vi "Run.vi"(8 "error in (no error)":errorcluster, 11 "IMD in":refnum<class "IMD.lvclass">) -> (0 "error out":errorcluster, 1 "Parameters":cluster{"Name":string, "Value":string}[](array[cluster]), 2 "Cancled":bool, 3 "IMD out":refnum<class "IMD.lvclass">)   [LabVIEW 2020, in "IMD.lvclass"]
doc: "This is the main test vi. It is here that the test is implemented."
uses:
  IMD.lvclass
  C:/Sandbox/RF Bench/Source Code/WiSpry Test Framework/Measurements/Measurement.lvclass
  Controls/Run states.ctl
  Devices/Controls/Change setting mode enum.ctl
  IMD.lvclass/IMD.ctl
  Instruments/Spectrum Analyzer/Spectrum Analyzer.lvclass/Spectrum Analyzer.ctl
  Measurement.lvclass/Measurement.ctl
  Path Control/Paths.ctl
  Support VI/Update parameters (single).vi
  Support VI/Update parameters (array).vi
  Measurement.lvclass
  Devices/Device.lvclass
  Instruments/Signal Generator/Signal Generator.lvclass
  Instruments/Spectrum Analyzer/Spectrum Analyzer.lvclass
  Devices/PIC-device/PIC-Device.lvclass
  XML Handler/XML Handler.lvclass
  Path Control/PathControl.lvclass
panel:
  in  "Power readings":dbl[](array[numeric])
  out "Current Delta Power [dB]":dbl
  out "Device Parameters":string
  out "Current Offset [Hz]":dbl format="%#_6p"
  out "Current Power [dBm]":dbl
  out "Current Frequency [Hz]":dbl format="%#_6p"
  out "Progress":u8(slide) scale=0.0..100.0
  in  "Cancel Button":bool
  out "XY Graph":cluster{dbl[], dbl[]}[](graph)
  out "Estimated finish time":timestamp format="%<%X>T"
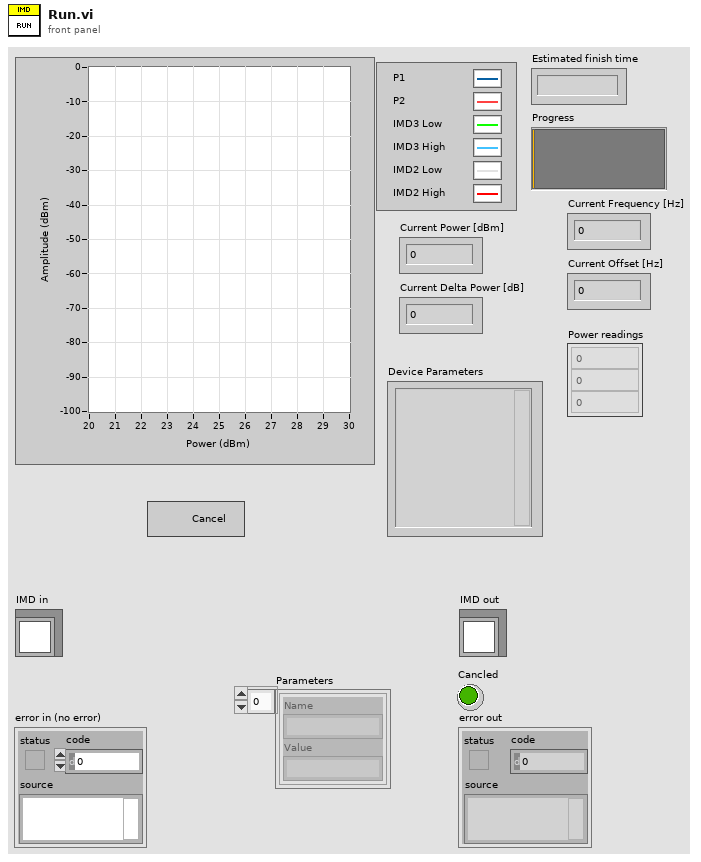
[diagram p1: front panel]
types:
  T1 = typedef "IMD.lvclass/Run states.ctl" = enum16{"Init", "Set Device", "Set Power", "Set Delta Power", "Set Frequency", "Set Offset", "Measure", "Done"}
  T2 = enum32{"Invalid", "Standard", "Closed", "Hidden", "Minimized", "Maximized"}
  T3 = typedef "PIC-Device.lvclass/Change setting mode enum.ctl" = enum16{"Init", "Next", "Reset"}
  T4 = typedef "IMD.lvclass/Config info.ctl" = cluster{"RBW":dbl, "VBW ":dbl, "Number of Averages":dbl, "Average On":bool, "Frequency (MHz)":string, "Offset Frequency (MHz)":string, "Power (dBm)":string, "Delta Power (dB)":string, "Uneven IMD":bool, "Loop order":T5, "Stop level":dbl, "IMD2":bool, "IMD3":bool}
  T5 = typedef "IMD.lvclass/Loop order.ctl" = enum16{"Device -> Power -> Frequency -> Offset", "Device -> Frequency -> Power -> Offset"}
  T6 = typedef "XML Handler.lvclass/Result Cluster.ctl" = cluster{"Name":string, "Value":string}
  T7 = typedef "PathControl.lvclass/Paths.ctl" = enum16{"SigGen 1 -> DUT", "SigGen 2 -> DUT", "SigGen 1 -> PM 1", "SigGen 1 -> PM 2", "DUT -> SA", "DUT -> PM 2", "VSG -> DUT", "SigGen 2 -> PM 1", "SigGen 2 -> PM 2"}
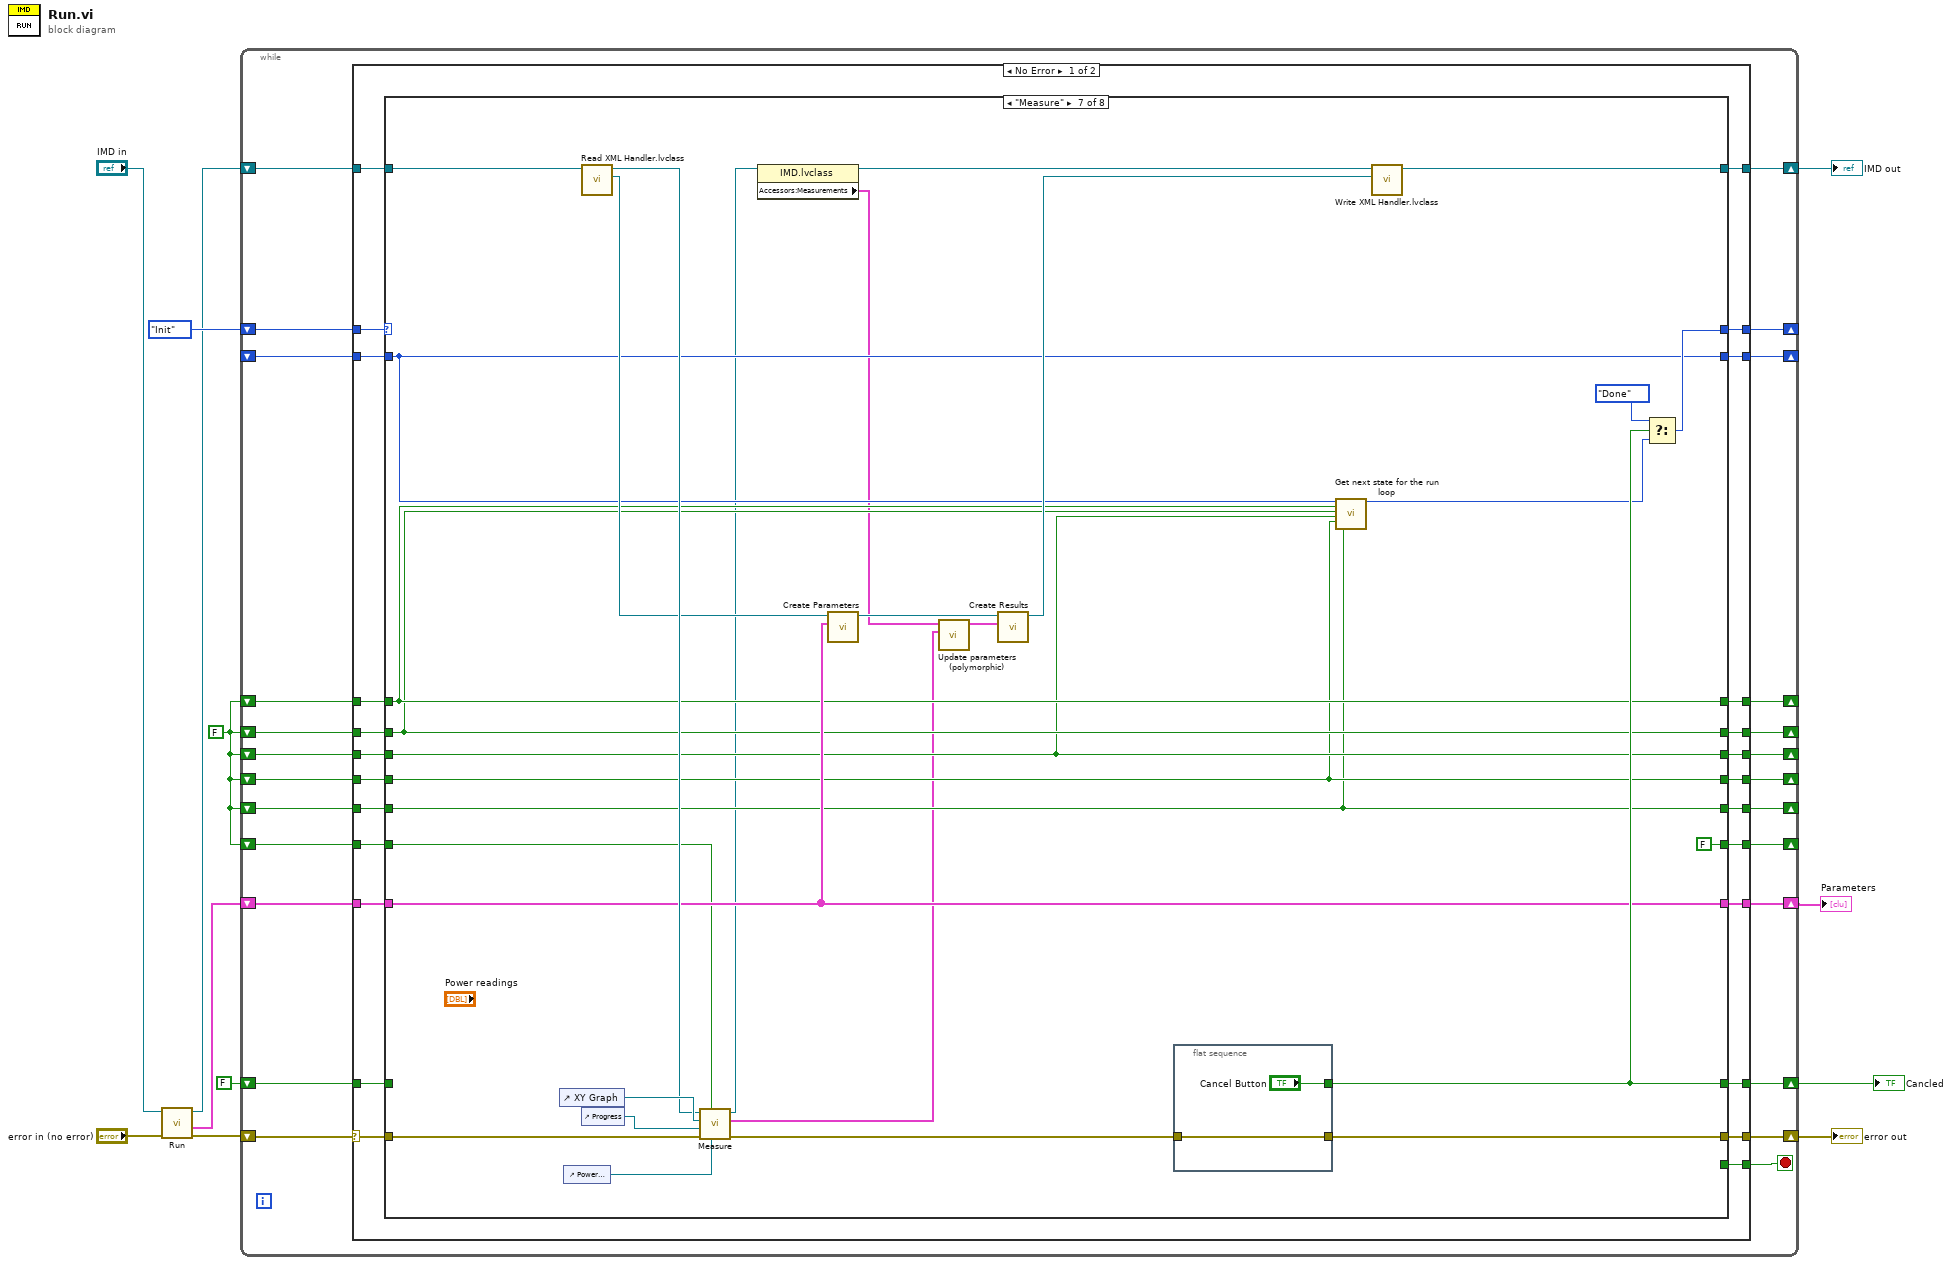
[diagram p0: block diagram]
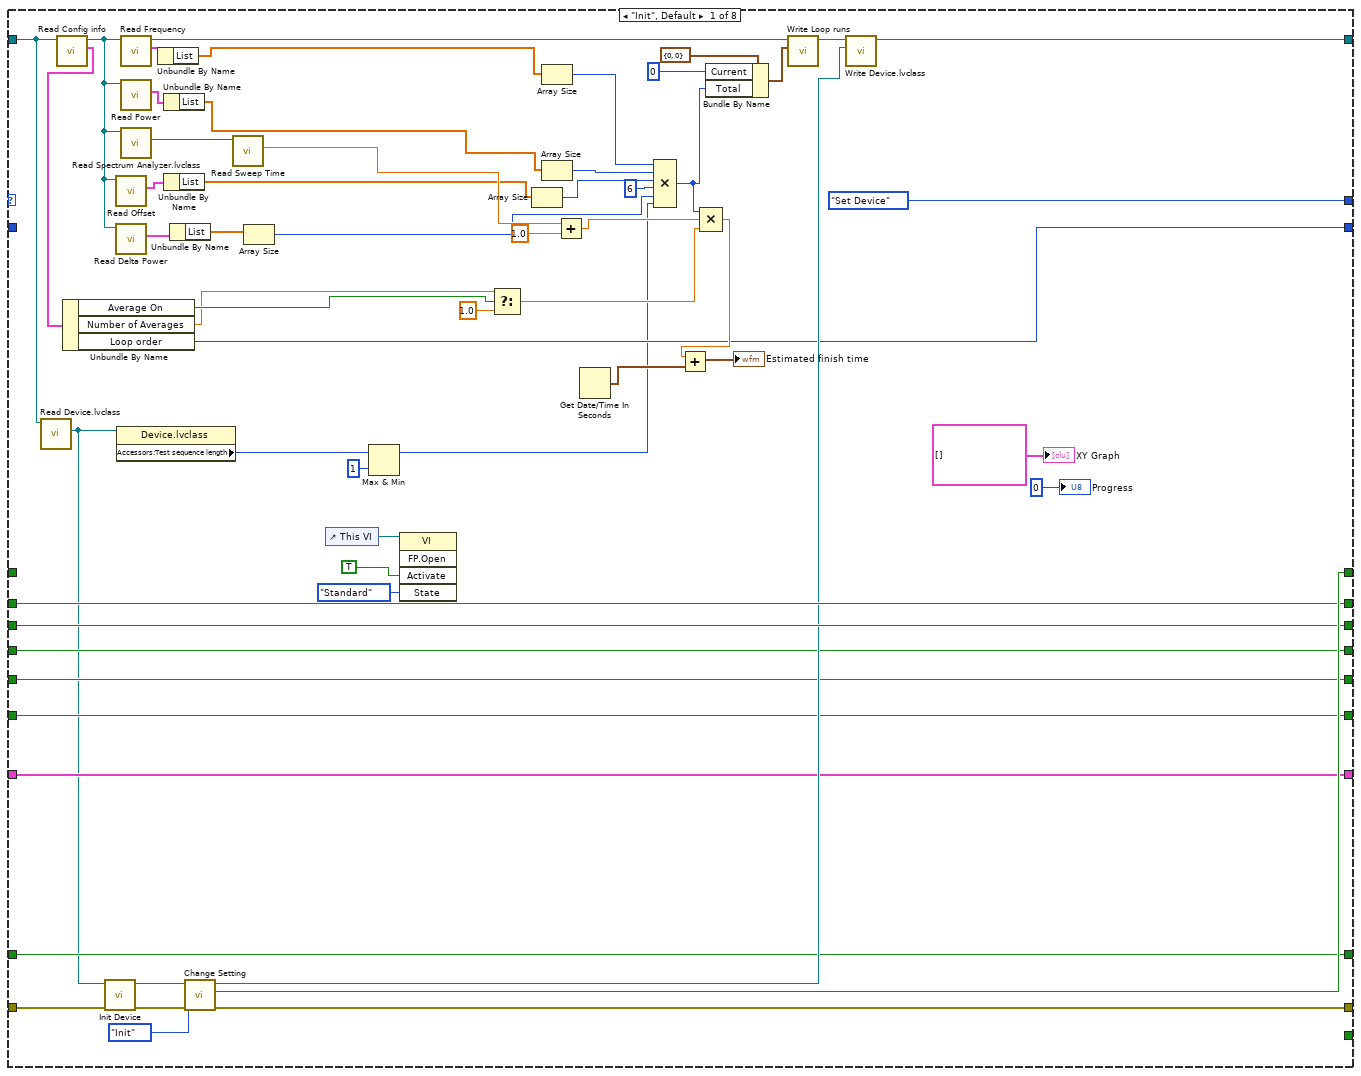
[diagram p2: hidden frame]
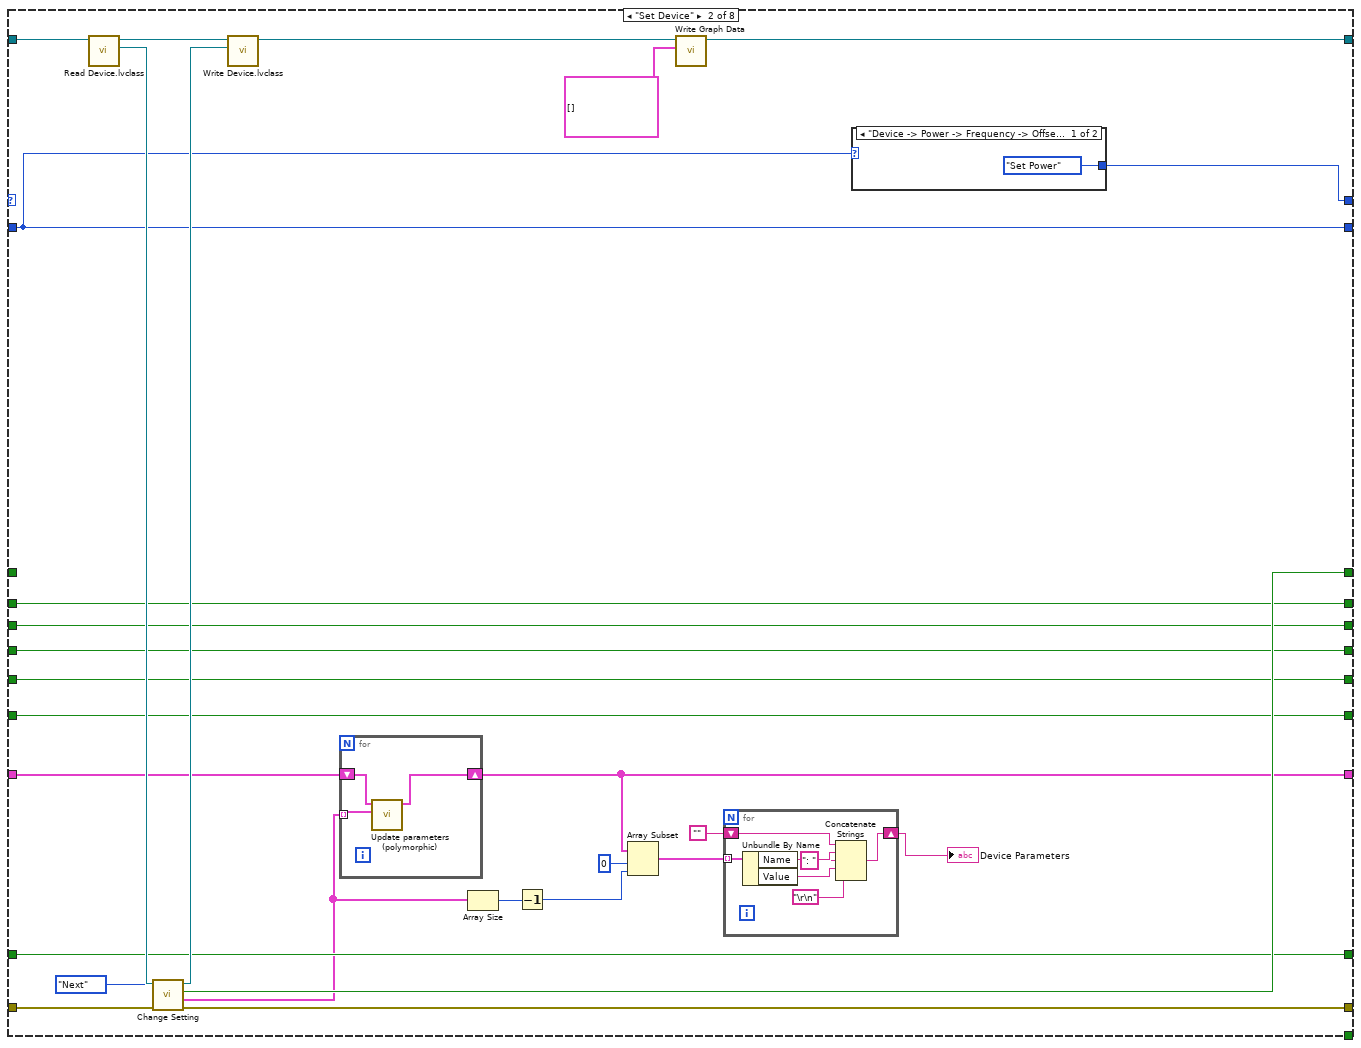
[diagram p3: hidden frame]
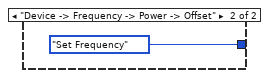
[diagram p4: hidden frame]
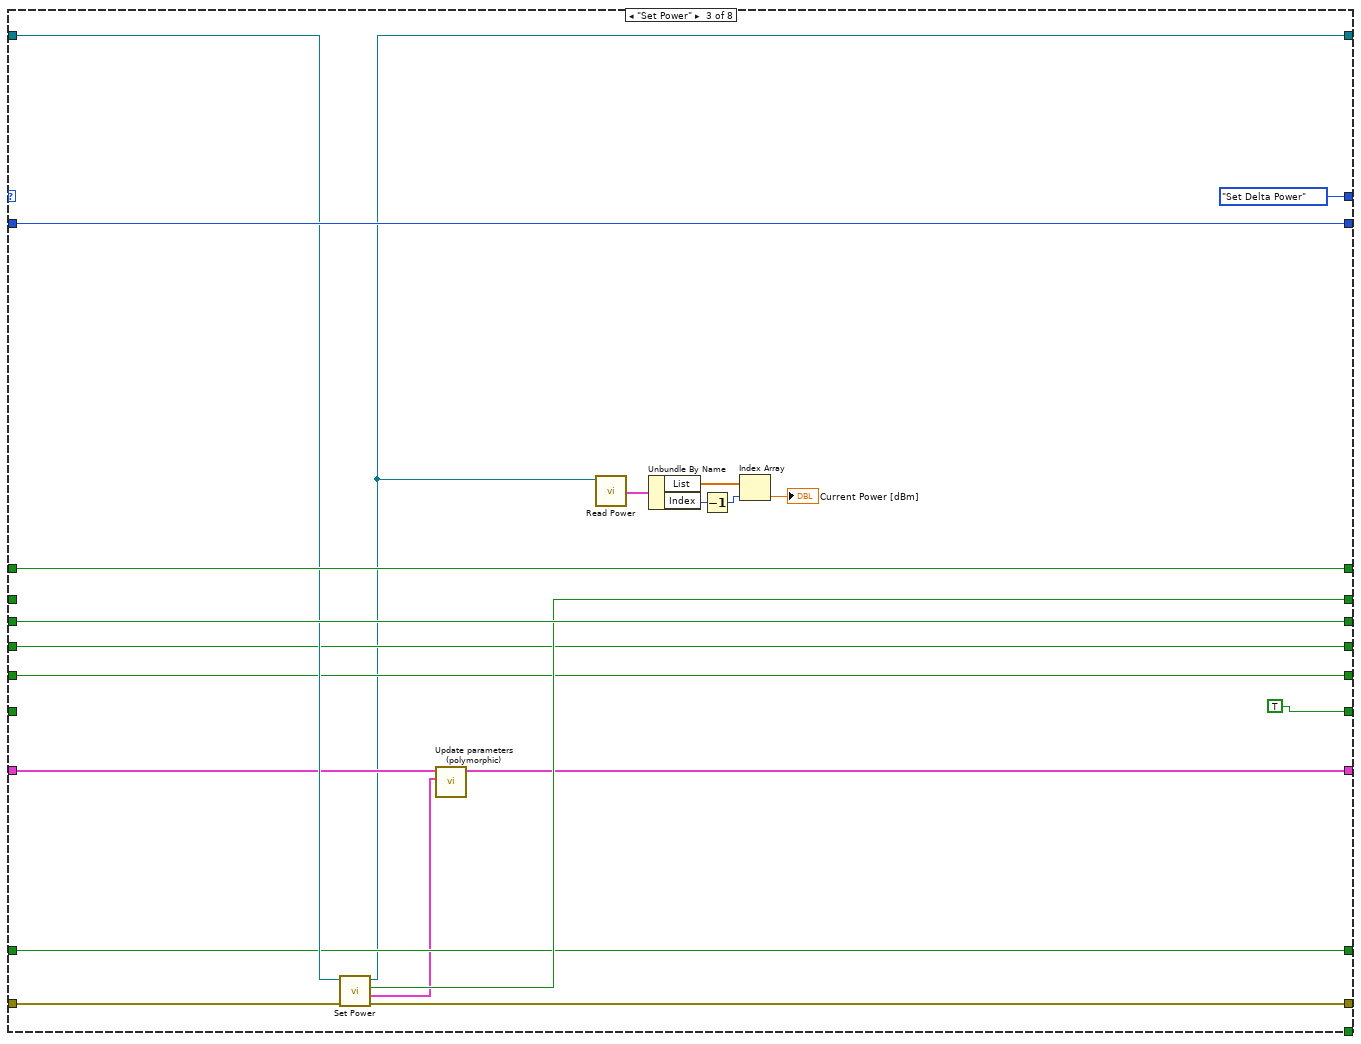
[diagram p5: hidden frame]
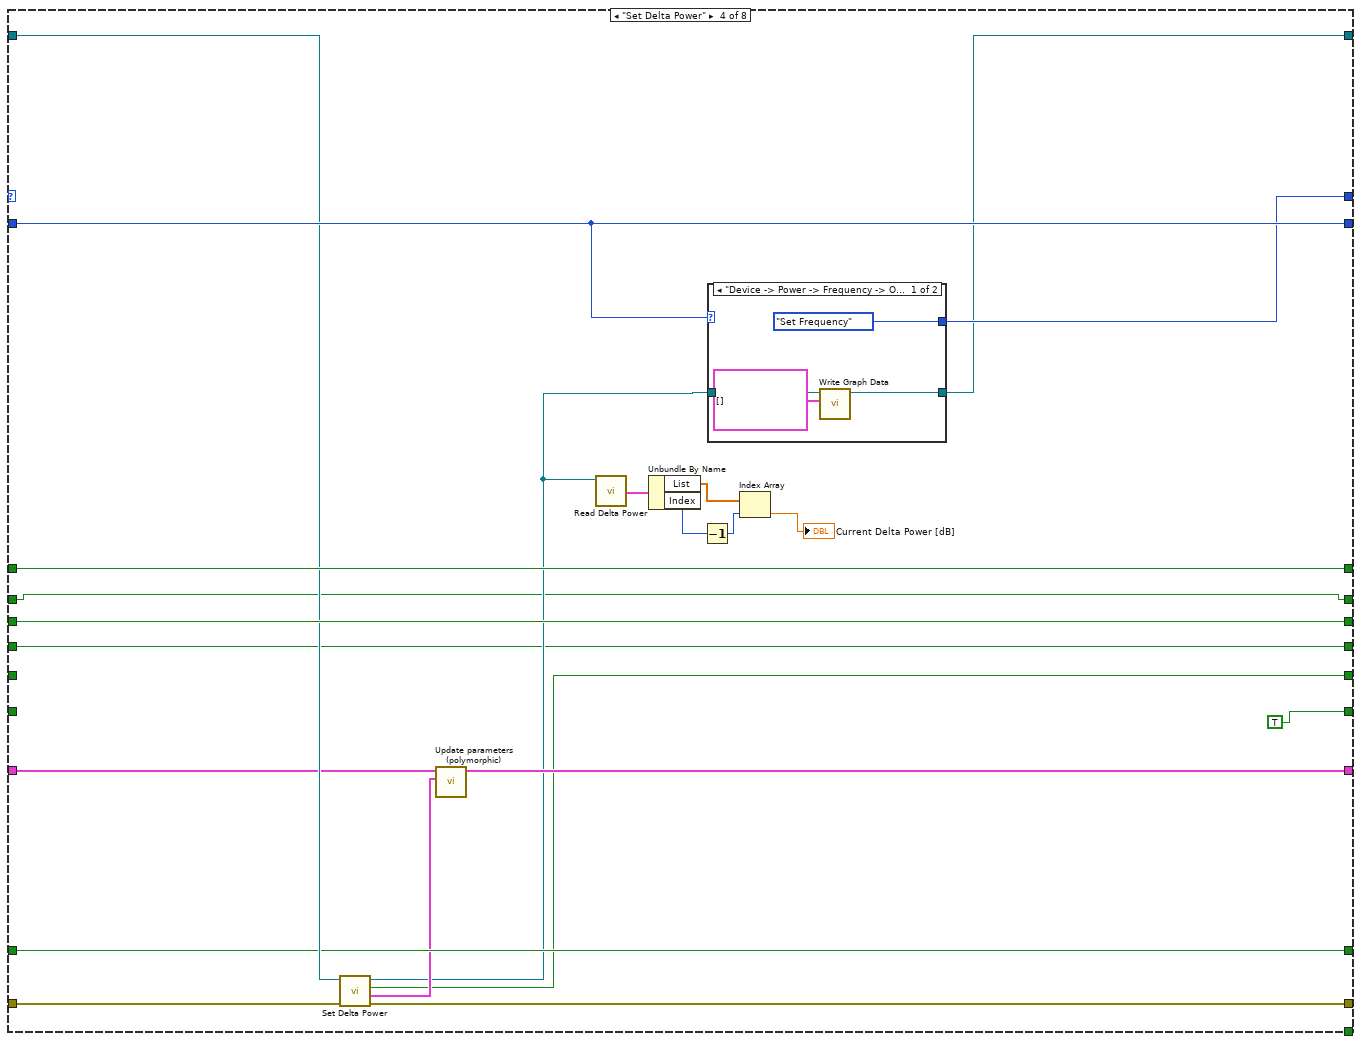
[diagram p6: hidden frame]
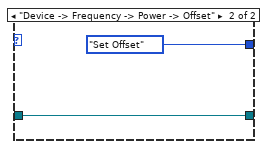
[diagram p7: hidden frame]
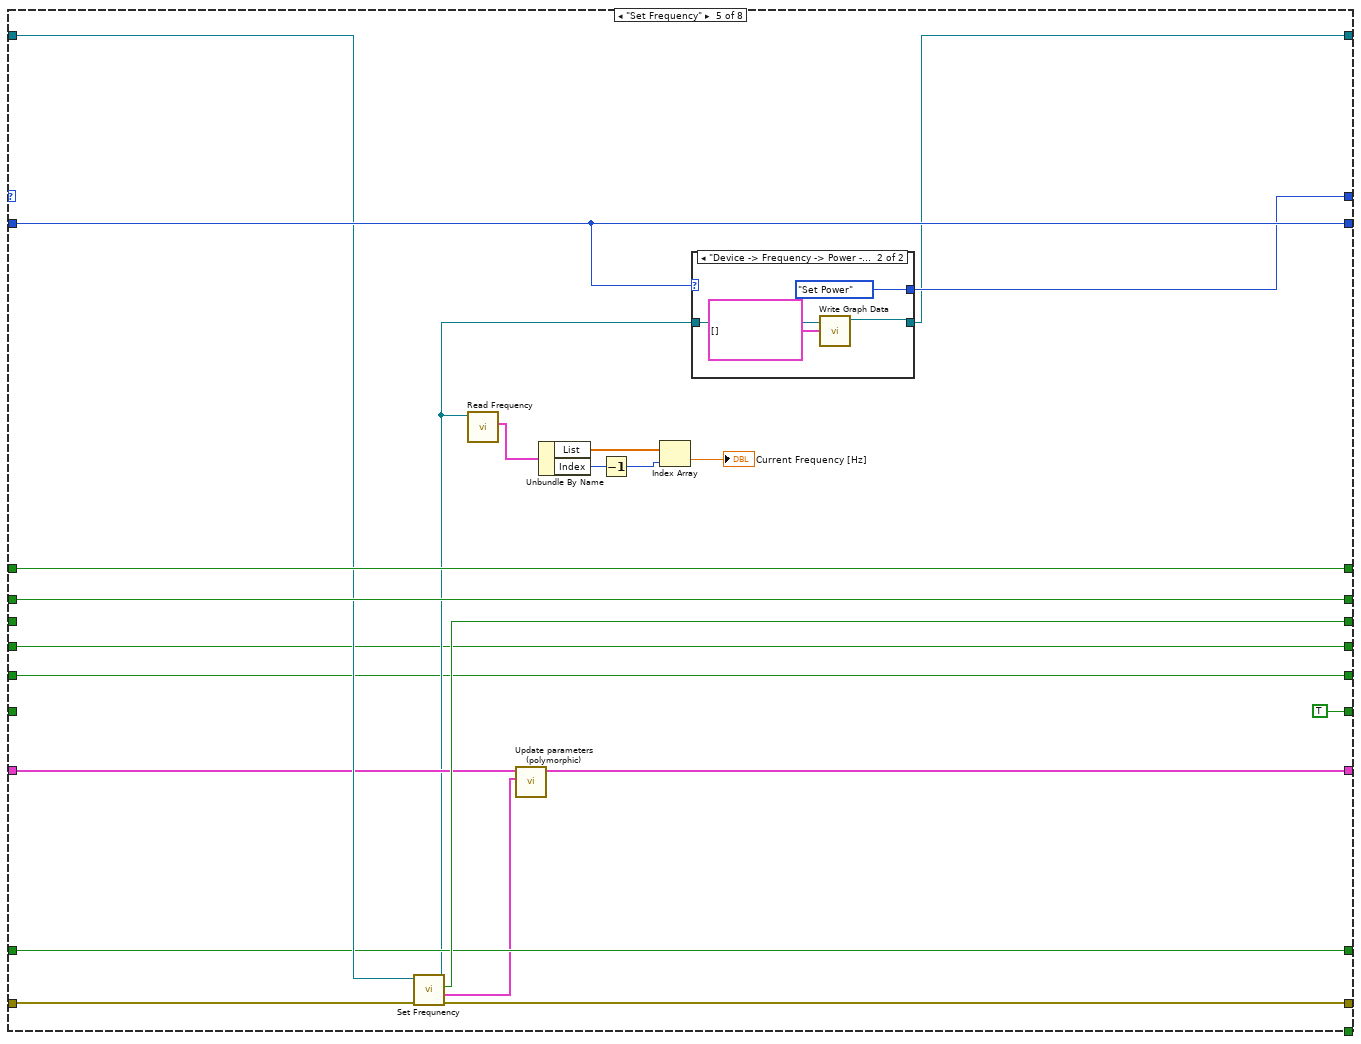
[diagram p8: hidden frame]
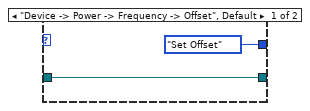
[diagram p9: hidden frame]
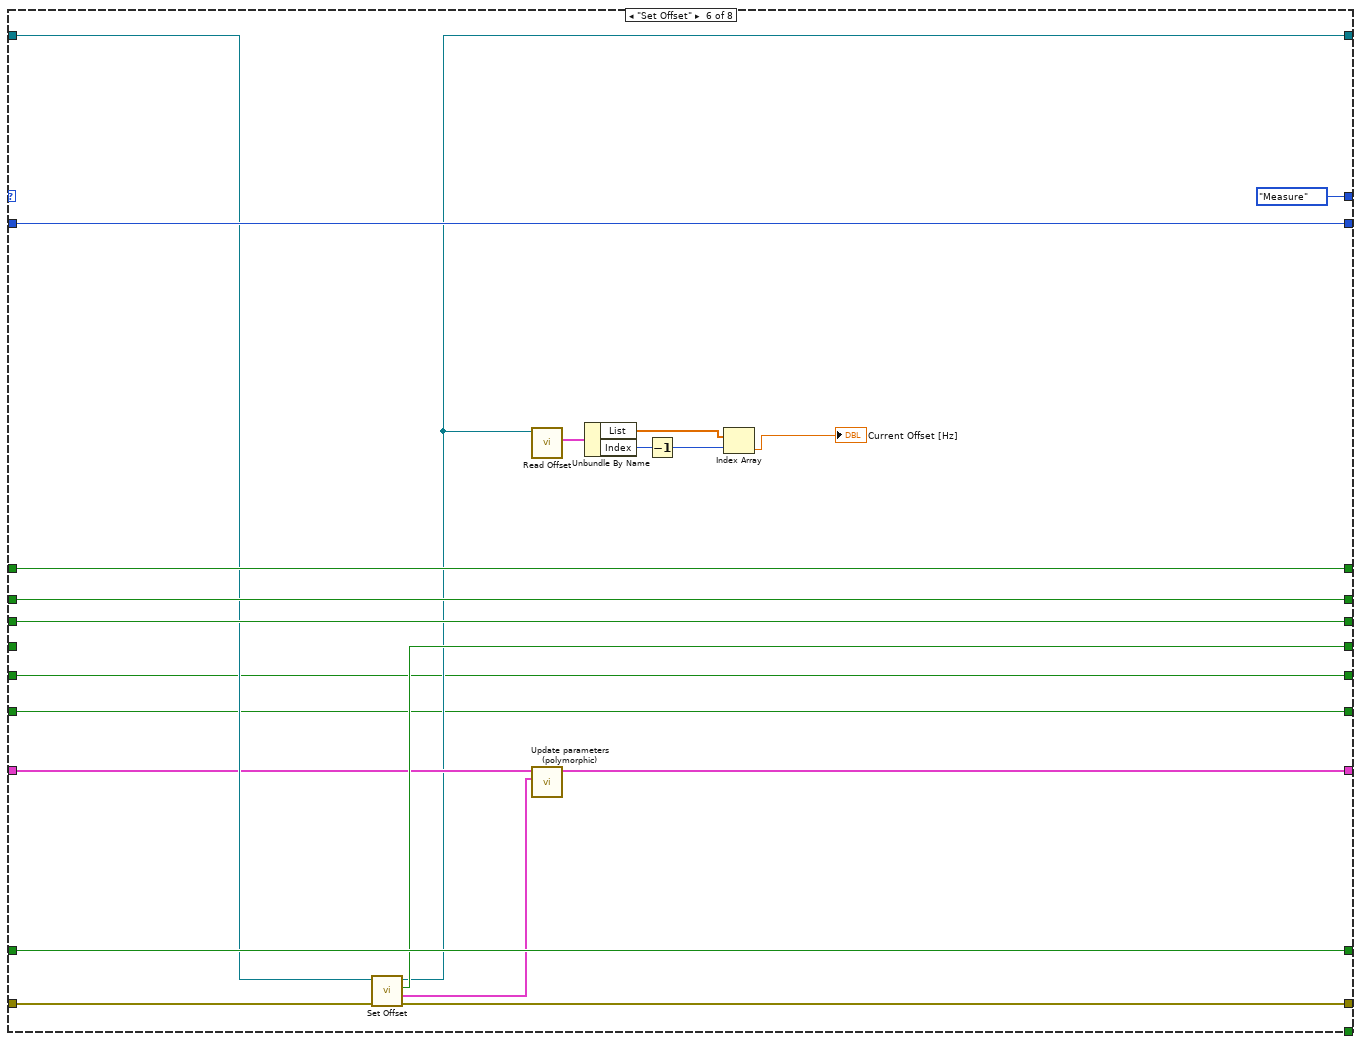
[diagram p10: hidden frame]
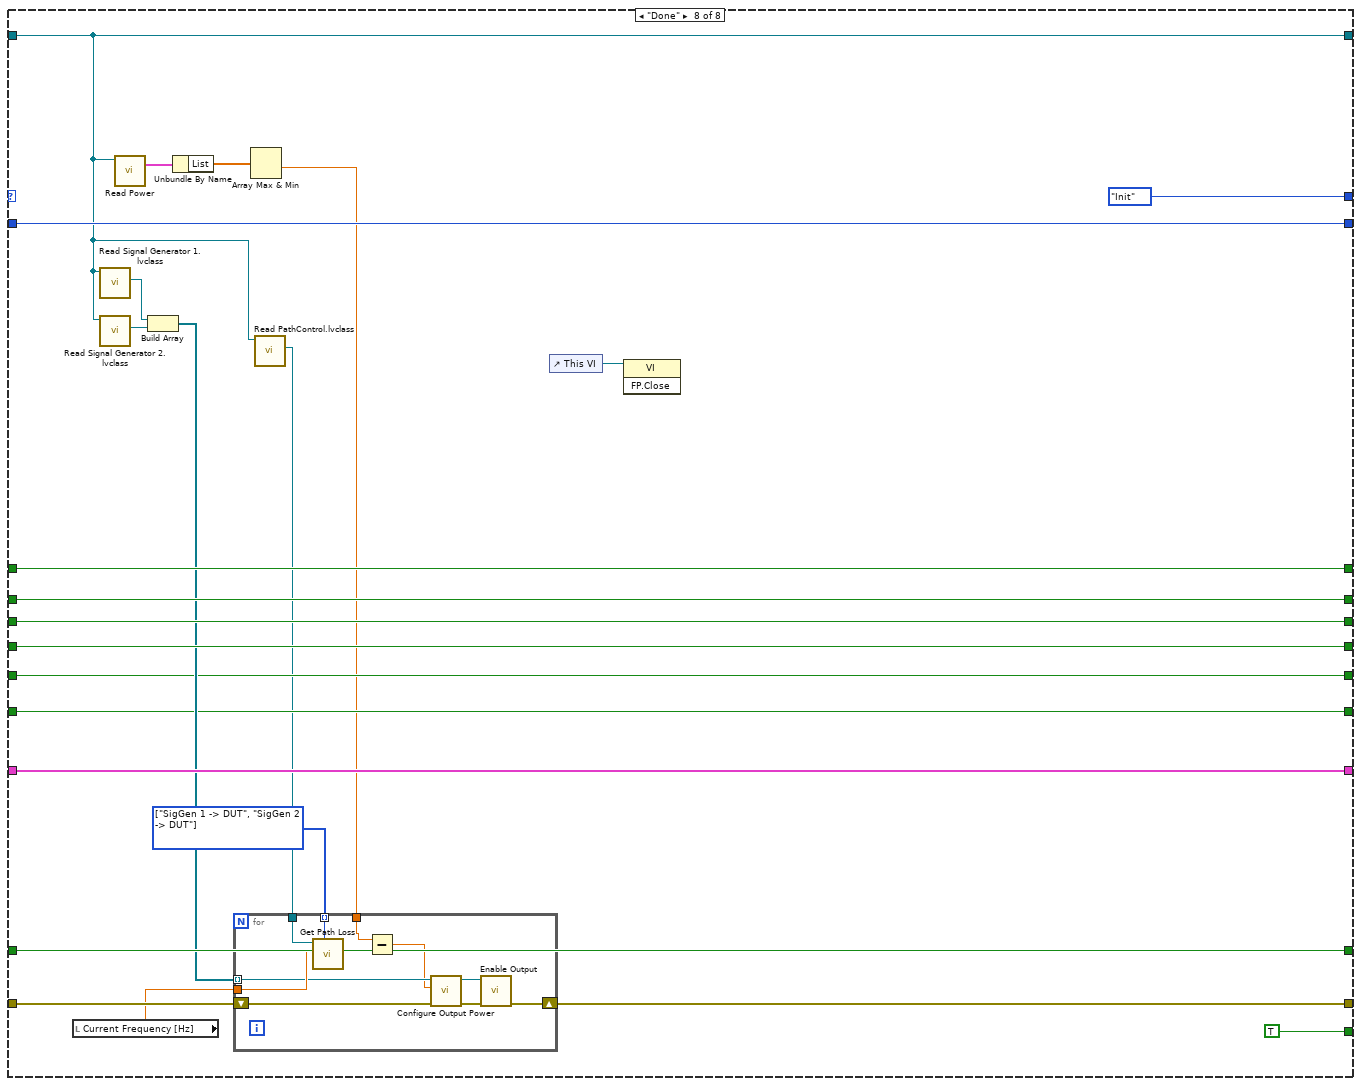
[diagram p11: hidden frame]
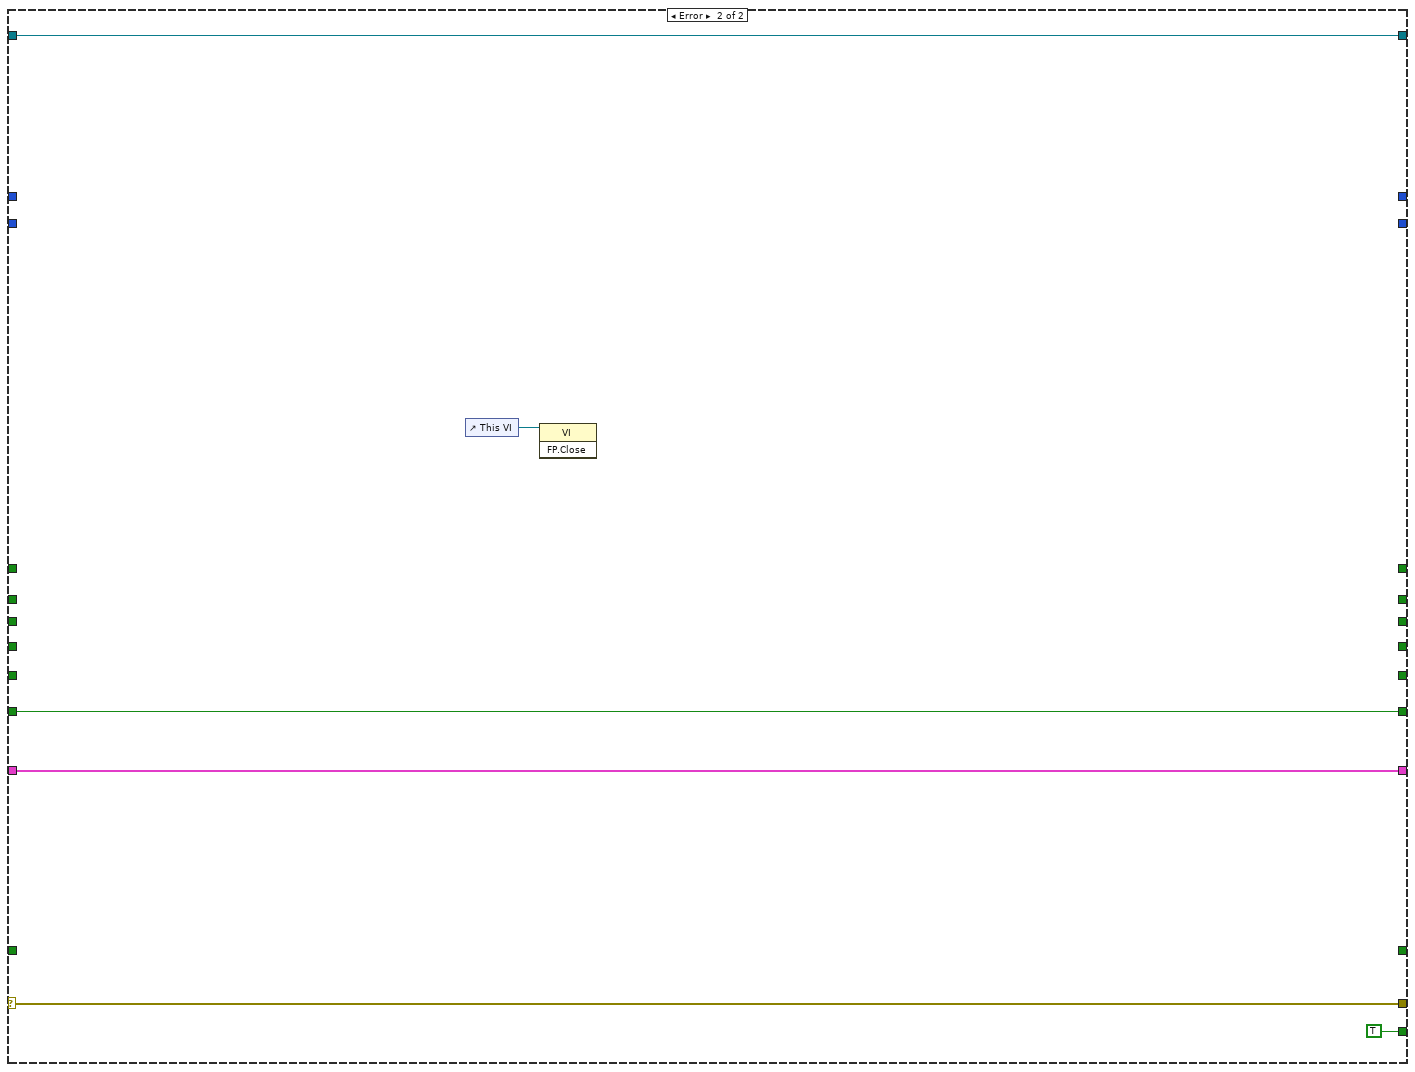
[diagram p12: hidden frame]
diagram:
  w7 = FALSE
  n1 = call-parent "Run.vi"("error in (no error)"="error in (no error)", "Measurements in"="IMD in") -> ("error out"=w4:errorcluster, "Parameters"=w3:cluster{"Name":string, "Value":string}[], "Measurements out"=w1:refnum<class "IMD.lvclass">)  [unwired: 6 in, 1 out]
  n2 = while {
    shift-right: [w32] -> w11
    shift-left: w4 -> [w37]
    shift-right: [w34] -> w12
    shift-left: w1 -> [w36]
    shift-right: [w29] -> _
    shift-left: Run_states."Init" ("Run states") -> [w35]
    shift-right: [w31] -> _
    shift-left: w7 -> [w30]
    shift-right: [w28] -> _
    shift-left: _ -> [w27]
    shift-right: [w24] -> _
    shift-left: w7 -> [w26]
    shift-right: [w23] -> _
    shift-left: w7 -> [w25]
    shift-right: [w22] -> w9
    shift-left: FALSE ("Cancel Button") -> [w21]
    shift-right: [w19] -> w6
    shift-left: w3 -> [w20]
    shift-right: [w17] -> _
    shift-left: w7 -> [w18]
    shift-right: [w15] -> _
    shift-left: w7 -> [w16]
    shift-right: [w13] -> _
    shift-left: w7 -> [w14]
    stop <- w33 stop-if-true
    n3 = case shown="No Error" w37 {
      selector: w37 -> [w59 w330]
      tunnel: w36 -> [w62 w331]
      tunnel: w35 -> [w61 _]
      tunnel: [w60 w331] -> w34
      tunnel: [w58 TRUE] -> w33
      tunnel: [w57 w330] -> w32
      tunnel: [w56 _] -> w31
      tunnel: w30 -> [w55 _]
      tunnel: [w54 _] -> w29
      tunnel: [w53 _] -> w28
      tunnel: w27 -> [w52 _]
      tunnel: w26 -> [w51 _]
      tunnel: w25 -> [w50 _]
      tunnel: [w49 _] -> w24
      tunnel: [w48 _] -> w23
      tunnel: [w47 _] -> w22
      tunnel: w21 -> [w46 _]
      tunnel: w20 -> [w45 w329]
      tunnel: [w44 w329] -> w19
      tunnel: w18 -> [w43 _]
      tunnel: [w42 _] -> w17
      tunnel: w16 -> [w41 _]
      tunnel: [w40 _] -> w15
      tunnel: w14 -> [w39 w328]
      tunnel: [w38 w328] -> w13
      frame No Error {
        n4 = case shown="\"Measure\"" w61 {
          tunnel: w62 -> [w112 w149 w178 w199 w227 w251 w261 w297]
          tunnel: [w79 w137 w164 w197 w224 w246 w285 w297] -> w60
          tunnel: w59 -> [w108 w146 w179 w200 w228 w253 w289 w307]
          tunnel: [_ _ _ _ _ _ _ TRUE] -> w58
          tunnel: [w104 w134 w175 w196 w223 w250 w283 w300] -> w57
          tunnel: [w102 w144 w182 w204 w232 w259 w274 w314] -> w56
          tunnel: w55 -> [_ _ w182 w204 w232 w259 w274 w314]
          tunnel: [Run_states."Set Device" ("Run states") w140 Run_states."Set Delta Power" ("Run states") w202 w230 Run_states."Measure" ("Run states") w280 Run_states."Init" ("Run states")] -> w54
          tunnel: [w84 w141 w181 w203 w231 w258 w275 w315] -> w53
          tunnel: w52 -> [_ w141 w181 w203 w231 w258 w275 w315]
          tunnel: w51 -> [w101 w143 _ w185 w229 w257 w273 w313]
          tunnel: w50 -> [w100 w142 w180 w201 _ w256 w272 w312]
          tunnel: [w101 w143 w177 w185 w229 w257 w273 w313] -> w49
          tunnel: [w100 w142 w180 w201 w226 w256 w272 w312] -> w48
          tunnel: [w94 w139 w176 w198 w225 w255 w282 w309] -> w47
          tunnel: w46 -> [w94 w139 w176 w198 w225 w255 _ w309]
          tunnel: w45 -> [w87 w133 w174 w195 w222 w249 w276 w306]
          tunnel: [w87 w126 w173 w194 w221 w248 w276 w306] -> w44
          tunnel: w43 -> [w78 w132 w166 w187 w213 _ w271 w305]
          tunnel: [w78 w132 w166 w187 w213 w252 w271 w305] -> w42
          tunnel: w41 -> [w75 w123 w165 _ w212 w240 w270 w302]
          tunnel: [w75 w123 w165 w184 w212 w240 w270 w302] -> w40
          tunnel: w39 -> [w70 w122 _ _ _ w239 w268 w301]
          tunnel: [w70 w122 TRUE TRUE TRUE w239 FALSE w301] -> w38
          frame "Init", Default {
            n5 = call "Read Device.lvclass.vi"("Measurements in"=w112) -> ("Device.lvclass"=w69:refnum<class "Device.lvclass">)  [unwired: 9 in, 1 out]
            n6 = call "Read Config info.vi"("IMD in"=w112) -> ("Config info"=w121:T4, "IMD out"=w74:refnum<class "IMD.lvclass">)  [unwired: 9 in]
            n7 = Unbundle By Name(w121) -> ("Average On"=w116:bool, "Number of Averages"=w115:dbl, "Loop order"=w84:T5)
            n8 = call-dynamic "Init Device.vi"("error in (no error)"=w108, "Device in"=w69) -> ("error out"=w105:errorcluster, "Device out"=w107:refnum<class "Device.lvclass">)  [unwired: 8 in]
            n9 = call "Read Offset.vi"("IMD in"=w74) -> ("Offset"=w83:cluster{"List":dbl[], "Index":i32, "Last":bool})  [unwired: 9 in, 1 out]
            n10 = call "Read Delta Power.vi"("IMD in"=w74) -> ("Delta Power"=w73:cluster{"List":dbl[], "Index":i32, "Last":bool})  [unwired: 9 in, 1 out]
            n11 = property class="Device.lvclass"(reference=w69) -> ("Accessors:Test sequence length"=w68:i32)  [unwired: 1 in, 2 out]
            n12 = call "Read Frequency.vi"("IMD in"=w74) -> ("Frequency"=w98:cluster{"List":dbl[], "Index":i32, "Last":bool}, "IMD out"=w93:refnum<class "IMD.lvclass">)  [unwired: 9 in]
            n13 = call "Read Power.vi"("IMD in"=w74) -> ("Power"=w96:cluster{"List":dbl[], "Index":i32, "Last":bool})  [unwired: 9 in, 1 out]
            n14 = call "Read Spectrum Analyzer.lvclass.vi"("IMD in"=w74) -> ("Spectrum Analyzer.lvclass"=w120:refnum<class "Spectrum Analyzer.lvclass">)  [unwired: 9 in, 1 out]
            n15 = Unbundle By Name(w98) -> ("List"=w97:dbl[])
            n16 = Unbundle By Name(w96) -> ("List"=w95:dbl[])
            n17 = Unbundle By Name(w83) -> ("List"=w82:dbl[])
            n18 = Unbundle By Name(w73) -> ("List"=w72:dbl[])
            n19 = call-dynamic "Change Setting.vi"("error in (no error)"=w105, "Change setting mode"=Change_setting_mode_enum."Init", "Device in"=w107) -> ("error out"=w104:errorcluster, "Last setting"=w102:bool, "Device out"=w99:refnum<class "Device.lvclass">)  [unwired: 5 in, 1 out]
            n20 = call "Read Sweep Time.vi"("Spectrum Analyzer in"=w120) -> ("Sweep Time"=w119:dbl)  [unwired: 9 in, 1 out]
            n21 = Array Size(array=w72) -> (size(s)=w71:i32)
            n22 = control-ref of="This VI"() -> (w65:refnum<vi>)
            n23 = Max & Min(x=w68, y=1) -> (max(x,y)=w67:i32)  [unwired: 1 out]
            n24 = invoke class="VI" method="FP.Open"(reference=w65, "Activate"=TRUE ("Activate?"), "State"=T2."Standard") -> ()  [unwired: 2 in, 5 out]
            n25 = Select(t=w115, s=w116, f=1.0) -> (s? t:f=w113:dbl)
            n26 = Array Size(array=w82) -> (size(s)=w81:i32)
            n27 = Array Size(array=w97) -> (size(s)=w110:i32)
            n28 = Array Size(array=w95) -> (size(s)=w109:i32)
            n29 = Add(x=w119, y=1.0) -> (x+y=w77:dbl)
            n30 = Get Date/Time In Seconds() -> (seconds since 1Jan1904=w118:timestamp)
            n31 = Compound Arithmetic op=MULTIPLY(w110, w109, w81, 6 ("value"), w71, w67) -> (w88:i32)
            n32 = Compound Arithmetic op=MULTIPLY(w88, w77, w113) -> (w111:dbl)
            n33 = Add(x=w111, y=w118) -> (x+y=→"Estimated finish time":timestamp)
            n34 = Bundle By Name(cluster=cluster{"Current":u32, "Total":u32} {"Current"=0, "Total"=0} ("Loop runs"), "Current"=u32 0, "Total"=w88) -> (w89:cluster{"Current":u32, "Total":u32})
            n35 = call "Write Loop runs.vi"("Loop runs"=w89, "Measurements in"=w93) -> ("Measurements out"=w92:refnum<class "IMD.lvclass">)  [unwired: 9 in]
            n36 = call "Write Device.lvclass.vi"("Device.lvclass"=w99, "Measurements in"=w92) -> ("Measurements out"=w79:refnum<class "IMD.lvclass">)  [unwired: 9 in]
            "XY Graph" <- cluster{dbl[], dbl[]}[] [] ("XY Graph")
            "Progress" <- u8 0 ("Progress")
          }
          frame "Set Device" {
            n37 = call "Read Device.lvclass.vi"("Measurements in"=w149) -> ("Device.lvclass"=w148:refnum<class "Device.lvclass">, "Measurements out"=w138:refnum<class "IMD.lvclass">)  [unwired: 9 in]
            n38 = call-dynamic "Change Setting.vi"("error in (no error)"=w146, "Change setting mode"=Change_setting_mode_enum."Next", "Device in"=w148) -> ("error out"=w134:errorcluster, "Changes"=w125:cluster{"Name":string, "Value":string}[], "Last setting"=w144:bool, "Device out"=w145:refnum<class "Device.lvclass">)  [unwired: 5 in]
            n39 = call "Write Device.lvclass.vi"("Device.lvclass"=w145, "Measurements in"=w138) -> ("Measurements out"=w135:refnum<class "IMD.lvclass">)  [unwired: 9 in]
            n40 = for {
              shift-right: [w158] -> w126
              shift-left: w133 -> [w159]
              tunnel: w125 -> [w157] mode=indexing
              n41 = call-poly "Update parameters (polymorphic).vi"("New Parameter"=w157, "Parameters"=w159) -> ("Parameters Out"=w158:cluster{"Name":string, "Value":string}[])  [unwired: 9 in]
            }
            n42 = Array Size(array=w125) -> (size(s)=w130:i32)
            n43 = Decrement(x=w130) -> (x-1=w127:i32)
            n44 = Array Subset(array=w126, index=0, length=w127) -> (w129:cluster{"Name":string, "Value":string}[])
            n45 = call "Write Graph Data.vi"("Graph Data"=cluster{"Array":dbl[], "Array":dbl[]}[] [], "IMD in"=w135) -> ("IMD out"=w137:refnum<class "IMD.lvclass">)  [unwired: 9 in]
            n46 = for {
              tunnel: w129 -> [w156] mode=indexing
              shift-right: [w150] -> w124
              shift-left: "" -> [w155]
              n47 = Unbundle By Name(w156) -> ("Name"=w154:string, "Value"=w152:string)
              n48 = Concatenate Strings(w155, w154, ": " ("string"), w152, "\r\n") -> (w150:string)
            }
            "Device Parameters" <- w124
            n49 = case shown="\"Device -> Power -> Frequency -> Offset\", Default" w141 {
              tunnel: [Run_states."Set Power" ("Run states") Run_states."Set Frequency" ("Run states")] -> w140
              frame "Device -> Power -> Frequency -> Offset", Default {
              }
              frame "Device -> Frequency -> Power -> Offset" {
              }
            }
          }
          frame "Set Power" {
            n50 = call "Set Power.vi"("error in (no error)"=w179, "IMD in"=w178) -> ("error out"=w175:errorcluster, "Parameter"=w172:cluster{"Name":string, "Value":string}, "Last Power?"=w177:bool, "IMD out"=w164:refnum<class "IMD.lvclass">)  [unwired: 6 in]
            n51 = call-poly "Update parameters (polymorphic).vi"("New Parameter"=w172, "Parameters"=w174) -> ("Parameters Out"=w173:cluster{"Name":string, "Value":string}[])  [unwired: 9 in]
            n52 = call "Read Power.vi"("IMD in"=w164) -> ("Power"=w171:cluster{"List":dbl[], "Index":i32, "Last":bool})  [unwired: 9 in, 1 out]
            n53 = Unbundle By Name(w171) -> ("List"=w169:dbl[], "Index"=w167:i32)
            n54 = Decrement(x=w167) -> (x-1=w168:i32)
            n55 = Index Array(array=w169, index=w168) -> (element=→"Current Power [dBm]":dbl)
          }
          frame "Set Delta Power" {
            n56 = call "Set Delta Power.vi"("error in (no error)"=w200, "IMD in"=w199) -> ("error out"=w196:errorcluster, "Parameter"=w193:cluster{"Name":string, "Value":string}, "Last Power?"=w184:bool, "IMD out"=w192:refnum<class "IMD.lvclass">)  [unwired: 6 in]
            n57 = call-poly "Update parameters (polymorphic).vi"("New Parameter"=w193, "Parameters"=w195) -> ("Parameters Out"=w194:cluster{"Name":string, "Value":string}[])  [unwired: 9 in]
            n58 = call "Read Delta Power.vi"("IMD in"=w192) -> ("Delta Power"=w191:cluster{"List":dbl[], "Index":i32, "Last":bool})  [unwired: 9 in, 1 out]
            n59 = Unbundle By Name(w191) -> ("List"=w190:dbl[], "Index"=w188:i32)
            n60 = Decrement(x=w188) -> (x-1=w189:i32)
            n61 = case shown="\"Device -> Power -> Frequency -> Offset\", Default" w203 {
              tunnel: [Run_states."Set Frequency" ("Run states") Run_states."Set Offset" ("Run states")] -> w202
              tunnel: w192 -> [w207 w209]
              tunnel: [w206 w209] -> w197
              frame "Device -> Power -> Frequency -> Offset", Default {
                n62 = call "Write Graph Data.vi"("Graph Data"=cluster{"Array":dbl[], "Array":dbl[]}[] [], "IMD in"=w207) -> ("IMD out"=w206:refnum<class "IMD.lvclass">)  [unwired: 9 in]
              }
              frame "Device -> Frequency -> Power -> Offset" {
              }
            }
            n63 = Index Array(array=w190, index=w189) -> (element=→"Current Delta Power [dB]":dbl)
          }
          frame "Set Frequency" {
            n64 = call "Set Frequnency.vi"("error in (no error)"=w228, "IMD in"=w227) -> ("error out"=w223:errorcluster, "Parameter"=w220:cluster{"Name":string, "Value":string}, "Last Frequency?"=w226:bool, "IMD out"=w219:refnum<class "IMD.lvclass">)  [unwired: 6 in]
            n65 = call "Read Frequency.vi"("IMD in"=w219) -> ("Frequency"=w218:cluster{"List":dbl[], "Index":i32, "Last":bool})  [unwired: 9 in, 1 out]
            n66 = call-poly "Update parameters (polymorphic).vi"("New Parameter"=w220, "Parameters"=w222) -> ("Parameters Out"=w221:cluster{"Name":string, "Value":string}[])  [unwired: 9 in]
            n67 = Unbundle By Name(w218) -> ("List"=w217:dbl[], "Index"=w216:i32)
            n68 = Decrement(x=w216) -> (x-1=w215:i32)
            n69 = Index Array(array=w217, index=w215) -> (element=→"Current Frequency [Hz]":dbl)
            n70 = case shown="\"Device -> Frequency -> Power -> Offset\"" w231 {
              tunnel: [Run_states."Set Offset" ("Run states") Run_states."Set Power" ("Run states")] -> w230
              tunnel: [w233 w236] -> w224
              tunnel: w219 -> [w233 w237]
              frame "Device -> Power -> Frequency -> Offset", Default {
              }
              frame "Device -> Frequency -> Power -> Offset" {
                n71 = call "Write Graph Data.vi"("Graph Data"=cluster{"Array":dbl[], "Array":dbl[]}[] [], "IMD in"=w237) -> ("IMD out"=w236:refnum<class "IMD.lvclass">)  [unwired: 9 in]
              }
            }
          }
          frame "Set Offset" {
            n72 = call "Set Offset.vi"("error in (no error)"=w253, "IMD in"=w251) -> ("error out"=w250:errorcluster, "Parameter"=w247:cluster{"Name":string, "Value":string}, "Last Offset?"=w252:bool, "IMD out"=w246:refnum<class "IMD.lvclass">)  [unwired: 6 in]
            n73 = call "Read Offset.vi"("IMD in"=w246) -> ("Offset"=w245:cluster{"List":dbl[], "Index":i32, "Last":bool})  [unwired: 9 in, 1 out]
            n74 = call-poly "Update parameters (polymorphic).vi"("New Parameter"=w247, "Parameters"=w249) -> ("Parameters Out"=w248:cluster{"Name":string, "Value":string}[])  [unwired: 9 in]
            n75 = Unbundle By Name(w245) -> ("List"=w244:dbl[], "Index"=w243:i32)
            n76 = Decrement(x=w243) -> (x-1=w241:i32)
            n77 = Index Array(array=w244, index=w241) -> (element=→"Current Offset [Hz]":dbl)
          }
          frame "Measure" {
            n78 = control-ref of="XY Graph"() -> (w287:refnum<vi>)
            n79 = control-ref of="Power readings"() -> (w260:refnum<vi>)
            n80 = call "Read XML Handler.lvclass.vi"("Measurements in"=w261) -> ("XML Handler.lvclass"=w278:refnum<class "XML Handler.lvclass">, "Measurements out"=w286:refnum<class "IMD.lvclass">)  [unwired: 9 in]
            n81 = control-ref of="Progress"() -> (w279:refnum<vi>)
            n82 = call "Measure.vi"("PM  results array Refnum"=w260, "Set Att"=w268, "error in (no error)"=w289, "Progress Ref"=w279, "XY Graph Reference"=w287, "IMD in"=w286) -> ("error out"=w284:errorcluster, "Results"=w266:T6[], "IMD out"=w264:refnum<class "IMD.lvclass">)  [unwired: 3 in]
            n83 = property class="IMD.lvclass"(reference=w264) -> (reference out=w263:refnum<class "IMD.lvclass">, "Accessors:Measurements"=w262:cluster{"Name":string, "Value":string}[])  [unwired: 1 in, 1 out]
            n84 = call "Create Parameters.vi"("Parameters"=w276, "XML Handler in"=w278) -> ("XML Handler out"=w277:refnum<class "XML Handler.lvclass">)  [unwired: 8 in, 1 out]
            n85 = call-poly "Update parameters (polymorphic).vi"("New Parameters"=w266, "Parameters"=w262) -> ("Parameters Out"=w265:cluster{"Name":string, "Value":string}[])  [unwired: 9 in]
            n86 = call "Create Results.vi"("Results"=w265, "XML Handler in"=w277) -> ("XML Handler out"=w288:refnum<class "XML Handler.lvclass">)  [unwired: 8 in, 1 out]
            n87 = flat-sequence {
              tunnel: w284 -> [w291]
              tunnel: [w291] -> w283
              tunnel: ["Cancel Button"] -> w282
              frame #0 {
              }
            }
            n88 = call "Get next state for the run loop.vi"("Loop order"=w275, "Last setting"=w274, "Last Power?"=w273, "Last Frequency?"=w272, "Last Offset?"=w271, "Last Power Delta?"=w270) -> ("Run states"=w269:T1)  [unwired: 13 in]
            n89 = call "Write XML Handler.lvclass.vi"("XML Handler.lvclass"=w288, "Measurements in"=w263) -> ("Measurements out"=w285:refnum<class "IMD.lvclass">)  [unwired: 9 in]
            n90 = Select(t=Run_states."Done", s=w282, f=w269) -> (s? t:f=w280:T1)
          }
          frame "Done" {
            w293 = T7[] [enum."SigGen 1 -> DUT", enum."SigGen 2 -> DUT"] items=["SigGen 1 -> DUT", "SigGen 2 -> DUT", "SigGen 1 -> PM 1", "SigGen 1 -> PM 2", "DUT -> SA", "DUT -> PM 2", "VSG -> DUT", "SigGen 2 -> PM 1", "SigGen 2 -> PM 2"]
            n91 = local read "Current Frequency [Hz]"() -> (w296:dbl)
            n92 = call "Read Signal Generator 1.lvclass.vi"("IMD in"=w297) -> ("Signal Generator 1.lvclass"=w308:refnum<class "Signal Generator.lvclass">)  [unwired: 9 in, 1 out]
            n93 = call "Read Signal Generator 2.lvclass.vi"("IMD in"=w297) -> ("Signal Generator.lvclass"=w303:refnum<class "Signal Generator.lvclass">)  [unwired: 9 in, 1 out]
            n94 = call "Read Power.vi"("IMD in"=w297) -> ("Power"=w299:cluster{"List":dbl[], "Index":i32, "Last":bool})  [unwired: 9 in, 1 out]
            n95 = Build Array(w308, w303) -> (w304:refnum<class "Signal Generator.lvclass">[])
            n96 = Unbundle By Name(w299) -> ("List"=w298:dbl[])
            n97 = Array Max & Min(array=w298) -> (min value=w294:dbl)  [unwired: 3 out]
            n98 = call "Read PathControl.lvclass.vi"("Measurements in"=w297) -> ("PathControl.lvclass"=w295:refnum<class "PathControl.lvclass">)  [unwired: 9 in, 1 out]
            n99 = for {
              tunnel: w304 -> [w322] mode=indexing
              shift-right: [w326] -> w300
              shift-left: w307 -> [w321]
              tunnel: w293 -> [w325] mode=indexing
              tunnel: w296 -> [w324]
              tunnel: w295 -> [w323]
              tunnel: w294 -> [w317]
              n100 = call "Get Path Loss.vi"("Path"=w325, "Frequency [Hz]"=w324, "PathControl in"=w323) -> ("Insertion Loss (dB)"=w318:dbl)  [unwired: 5 in, 3 out]
              n101 = Subtract(x=w317, y=w318) -> (x-y=w316:dbl)
              n102 = call-dynamic "Configure Output Power.vi"("error in (no error)"=w321, "Output Power [dBm]"=w316, "Signal Generator in"=w322) -> ("error out"=w319:errorcluster, "Signal Generator out"=w320:refnum<class "Signal Generator.lvclass">)  [unwired: 7 in]
              n103 = call-dynamic "Enable Output.vi"("error in (no error)"=w319, "Signal Generator in"=w320) -> ("error out"=w326:errorcluster)  [unwired: 8 in, 1 out]
            }
            n104 = control-ref of="This VI"() -> (w292:refnum<vi>)
            n105 = invoke class="VI" method="FP.Close"(reference=w292) -> ()  [unwired: 2 in, 3 out]
          }
        }
      }
      frame Error {
        n106 = control-ref of="This VI"() -> (w327:refnum<vi>)
        n107 = invoke class="VI" method="FP.Close"(reference=w327) -> ()  [unwired: 2 in, 3 out]
      }
    }
  }
  "error out" <- w11
  "IMD out" <- w12
  "Cancled" <- w9
  "Parameters" <- w6
